vi "MoveSampleAndSave.vi"() -> ()   [LabVIEW 2017]
uses:
  <vilib>/Analysis/baseanly.llb/Mean (DBL).vi
  <vilib>/Analysis/NI_AALBase.lvlib
panel:
  out "5V Indicator 3":bool
  in  "Calibration Constant 2":dbl
  in  "Forward/Reverse 2":bool
  in  "Distance/Sample 2":dbl
  in  "Calibration Constant":dbl
  in  "Offset (V)":dbl
  in  "Distance/Sample":dbl
  in  "Axis#":i16 min=0 max=2 step=1
  in  "Forward/Reverse":bool
  out "5V Indicator":bool
  in  "Total Distance (mm) (X-Axis)":dbl
  # "Y AXIS"
  # "PITOT TUBE"
  # "X AXIS"
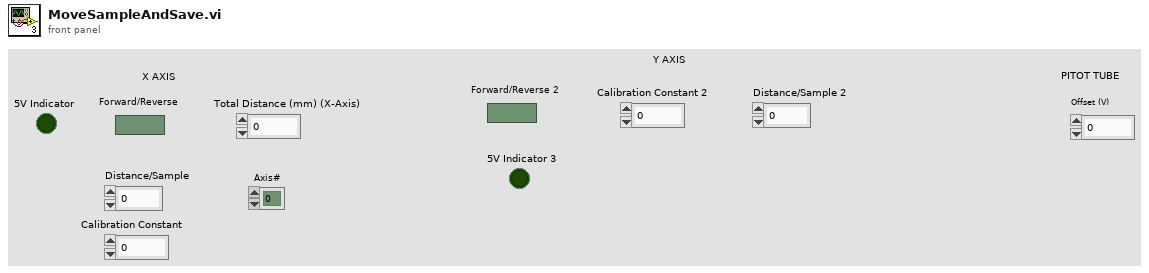
[diagram p1: front panel]
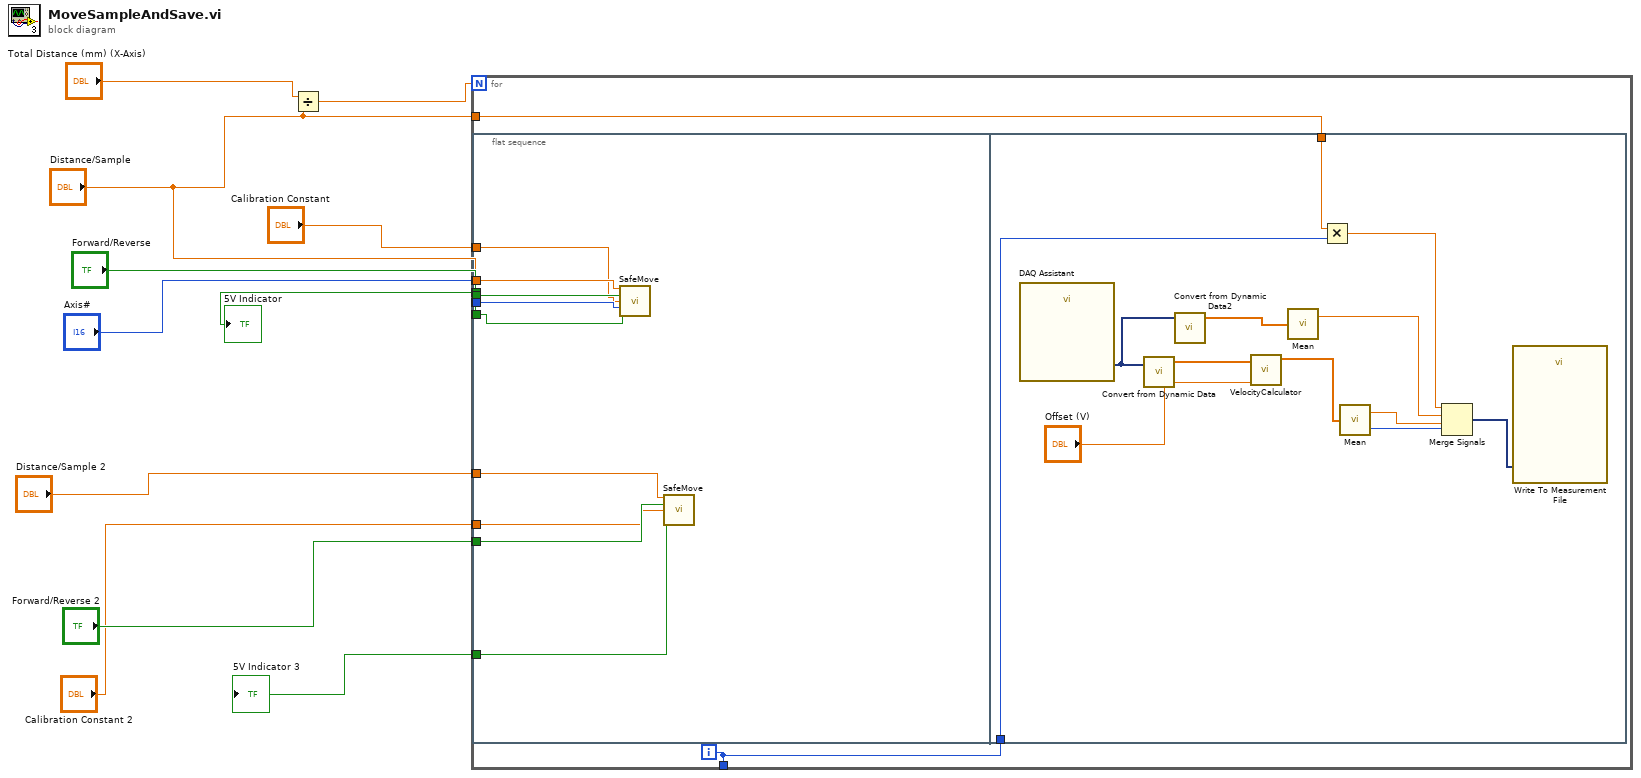
[diagram p0: block diagram]
diagram:
  n1 = Divide(x="Total Distance (mm) (X-Axis)", y="Distance/Sample") -> (x/y=w7:dbl)
  n2 = for {
    N: w7 -> [_]
    tunnel: [w17] -> w11
    tunnel: "Forward/Reverse" -> [w19]
    tunnel: "Axis#" -> [w18]
    tunnel: "Distance/Sample" -> [w22]
    tunnel: [w21] -> _
    tunnel: "Distance/Sample" -> [w20]
    tunnel: "Calibration Constant" -> [w16]
    tunnel: "Distance/Sample 2" -> [w13]
    tunnel: "Forward/Reverse 2" -> [w15]
    tunnel: "Calibration Constant 2" -> [w14]
    tunnel: [w12] -> w1
    i -> [w21]
    n3 = flat-sequence {
      tunnel: w19 -> [_]
      tunnel: w22 -> [w31]
      tunnel: w19 -> [w30]
      tunnel: w18 -> [w29]
      tunnel: [w28] -> w17
      tunnel: w16 -> [w27]
      tunnel: w15 -> [w26]
      tunnel: w14 -> [w25]
      tunnel: w13 -> [w24]
      tunnel: [w23] -> w12
      tunnel: w21 -> [w34]
      tunnel: w20 -> [w33]
      frame #0 {
        n4 = call "SafeMove.vi"("Total Distance (mm)"=w31, "Forward/Reverse"=w30, "Calibration Constant"=w27, "Axis#"=w29) -> ("5V Indicator"=w28:bool)  [unwired: 11 in]
        n5 = call "SafeMove.vi"("Total Distance (mm)"=w24, "Forward/Reverse"=w26, "Calibration Constant"=w25) -> ("5V Indicator"=w23:bool)  [unwired: 12 in]
      }
      frame #1 {
        n6 = call "DAQ Assistant"() -> ("data"=w37:dynamicdata)  [unwired: 17 in, 2 out]
        n7 = call "Convert from Dynamic Data"("Dynamic Data Type"=w37) -> ("Array"=w43:dbl[])  [unwired: 3 in]
        n8 = call "Convert from Dynamic Data2"("Dynamic Data Type"=w37) -> ("Array"=w36:dbl[])  [unwired: 3 in]
        n9 = call "VelocityCalculator.vi"("Offset (V)"="Offset (V)", "Voltage Input"=w43) -> ("Veloctiy Output [m/s]"=w42:dbl[])  [unwired: 9 in]
        n10 = call-poly <vilib>:"Mean.vi"("X"=w36) -> ("mean"=w35:dbl)  [unwired: 1 out]
        n11 = Multiply(x=w33, y=w34) -> (x*y=w32:dbl)
        n12 = call-poly <vilib>:"Mean.vi"("X"=w42) -> ("mean"=w40:dbl, "error"=w39:i32)
        n13 = Merge Signals(w32, w35, w40, w39) -> (w41:dynamicdata)
        n14 = call "Write To Measurement File"("Signals"=w41) -> ()  [unwired: 16 in, 3 out]
      }
    }
  }
  "5V Indicator" <- w11
  "5V Indicator 3" <- w1
